vi "create_full_request_data.vi"(0 "llm_openai_embedding in":refnum<class "llm_gemini_embedding.lvclass">, 5 "data":refnum<class "abstract_message_base.lvclass">[](array[class]), 11 "error in (no error)":errorcluster) -> (4 "llm_openai_embedding out":refnum<class "llm_gemini_embedding.lvclass">, 6 "request_data":T1[](array[typedef]), 15 "error out":errorcluster)   [LabVIEW 2020, in "llm_gemini_embedding.lvclass"]
uses:
  llm_gemini_embedding.lvclass
  abstract_message_base/abstract_message_base.lvclass
  utils/request_Data.ctl
  llm_gemini_embedding.lvclass/llm_gemini_embedding.ctl
  message_text/message_text.lvclass
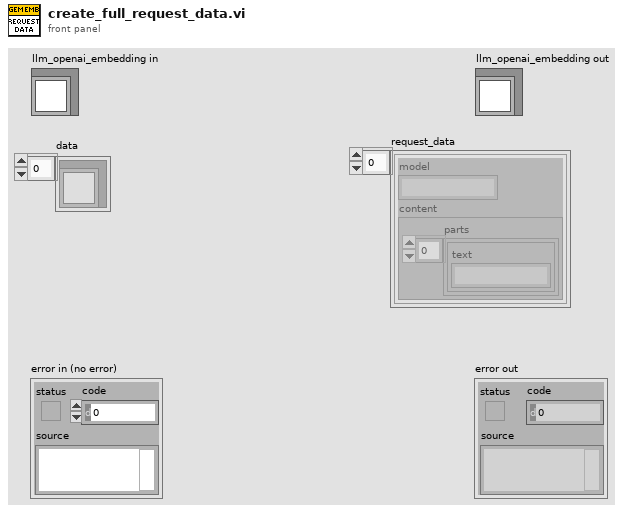
[diagram p1: front panel]
types:
  T1 = typedef "llm_gemini_embedding.lvclass/request_Data.ctl" = cluster{"model":string, "content":cluster{"parts":cluster{"text":string}[]}}
  T2 = typedef "message_text.lvclass/message.ctl" = cluster{"role":string, "content":string[]}
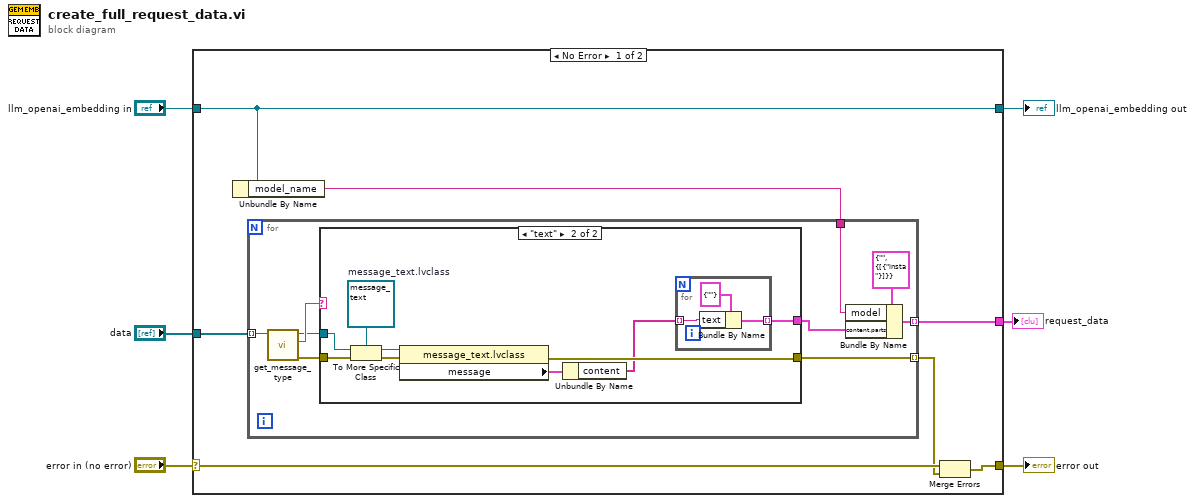
[diagram p0: block diagram]
diagram:
  n1 = case shown="No Error" "error in (no error)" {
    selector: "error in (no error)" -> [w13 w37]
    tunnel: [w8 w37] -> w5
    tunnel: [w11 w36] -> w3
    tunnel: "llm_openai_embedding in" -> [w11 w36]
    tunnel: "data" -> [w12 _]
    tunnel: [w9 _] -> w1
    frame No Error {
      n2 = Unbundle By Name(w11) -> ("model_name"=w10:string)
      n3 = for {
        tunnel: w12 -> [w22] mode=indexing
        tunnel: [w18] -> w7 mode=indexing
        tunnel: w10 -> [w17]
        tunnel: [w16] -> w9 mode=indexing
        n4 = call-dynamic "get_message_type.vi"("abstract_message_base in"=w22) -> ("error out"=w19:errorcluster, "Type"=w21:string, "abstract_message_base out"=w20:refnum<class "abstract_message_base.lvclass">)  [unwired: 8 in]
        n5 = case shown="\"text\"" w21 {
          tunnel: w20 -> [_ w31]
          tunnel: w19 -> [w23 w32]
          tunnel: [w23 w27] -> w18
          tunnel: [_ w25] -> w14
          frame Default {
          }
          frame "text" {
            w30 = refnum<class "message_text.lvclass"> refnum  # message_text.lvclass
            n6 = To More Specific Class(target class=w30, reference=w31, error in=w32) -> (specific class reference=w29:refnum<class "message_text.lvclass">, error out=w28:errorcluster)
            n7 = property class="message_text.lvclass"(reference=w29, error in=w28) -> (error out=w27:errorcluster, "message"=w26:T2)  [unwired: 1 out]
            n8 = Unbundle By Name(w26) -> ("content"=w24:string[])
            n9 = for {
              tunnel: [w34] -> w25 mode=indexing
              tunnel: w24 -> [w33] mode=indexing
              n10 = Bundle By Name(cluster=cluster{"text":string} {"text"=""} ("content.parts"), "text"=w33) -> (w34:cluster{"text":string})
            }
          }
        }
        n11 = Bundle By Name(cluster=T1 {"model"="", "content"={"parts"=[{"text"="insta"}]}} ("request data"), "model"=w17, "content.parts"=w14) -> (w16:T1)
      }
      n12 = Merge Errors(w13, w7) -> (w8:errorcluster)
    }
    frame Error {
    }
  }
  "error out" <- w5
  "llm_openai_embedding out" <- w3
  "request_data" <- w1
